vi "NI Analog.vi"(8 "error in (no error)":errorcluster, 11 "Message Queues":T1) -> (0 "error out":errorcluster, 3 "Message Queue out":refnum<queue>)   [LabVIEW 2014]
uses:
  support/Message Queue/All Message Queues.ctl
  support/Message Queue/Message Cluster.ctl
  Analog data.ctl
  Analog Input Cluster.ctl
  Analog Result Cluster.ctl
  <vilib>/DAQmx/write.llb/DAQmx Write (Analog DBL 1Chan 1Samp).vi
  <vilib>/DAQmx/read.llb/DAQmx Read (Analog 1D DBL 1Chan NSamp).vi
  <vilib>/DAQmx/read.llb/DAQmx Read (Analog 2D DBL NChan NSamp).vi
  support/Message Queue/Enqueue Message (Single).vi
  <vilib>/DAQmx/miscellaneous.llb/DAQmx Fill In Error Info.vi
  support/Message Queue/Lossy Enqueue Message (Single).vi
  <vilib>/Utility/error.llb/Error Cluster From Error Code.vi
  <vilib>/ErrorRing/Error Ring.xnode
  support/Message Queue/Message Queue.lvlib
panel:
  out "Port Write Time [ms] 2":u32
  out "Port Write Time [ms]":u32
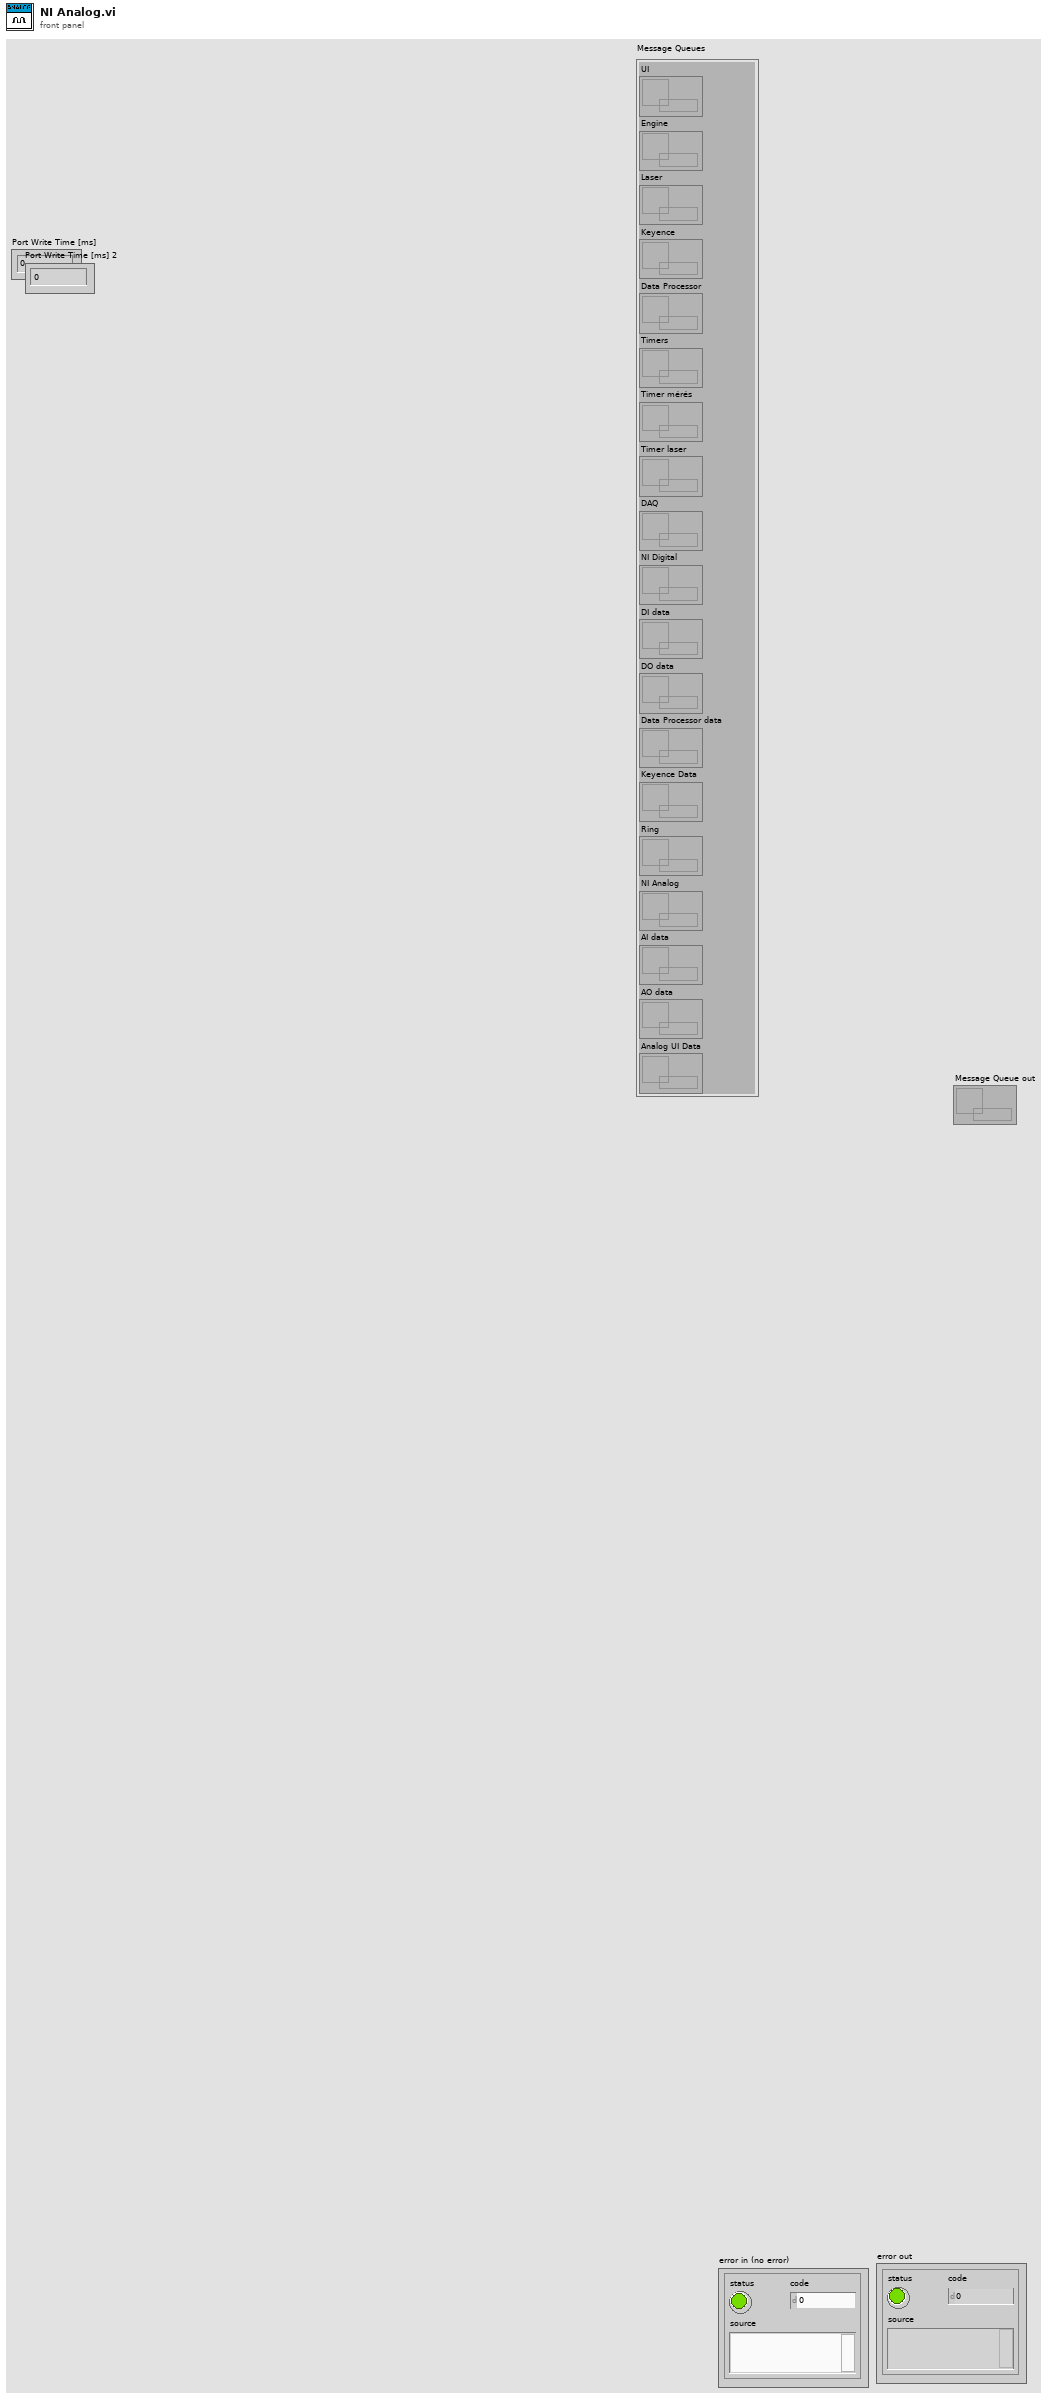
[diagram p1: front panel]
types:
  T1 = typedef "Message Queue.lvlib/All Message Queues.ctl" = cluster{"UI":refnum<queue>, "Engine":refnum<queue>, "Laser":refnum<queue>, "Keyence":refnum<queue>, "Data Processor":refnum<queue>, "Timers":refnum<queue>, "Timer mérés":refnum<queue>, "Timer laser":refnum<queue>, "DAQ":refnum<queue>, "NI Digital":refnum<queue>, "DI data":refnum<queue>, "DO data":refnum<queue>, "Data Processor data":refnum<queue>, "Keyence Data":refnum<queue>, "Ring":refnum<queue>, "NI Analog":refnum<queue>, "AI data":refnum<queue>, "AO data":refnum<queue>, "Analog UI Data":refnum<queue>}
  T2 = typedef "Analog data.ctl" = cluster{"URref":refnum<k21>, "UR":refnum<k21>, "UNTC":refnum<k21>, "UISOL":refnum<k21>, "TEMP":refnum<k21>, "dUref":refnum<k21>, "dU_":refnum<k21>, "UCTRL":refnum<k21>, "U48":refnum<k21>, "NI analog":refnum<k21>}
  T3 = typedef "Analog Input Cluster.ctl" = cluster{"NI-6221":cluster{"Sensor":dbl, "Uref":dbl, "Temperature":dbl, "Uisol":dbl, "NTC":dbl, "U48":dbl, "U15":dbl}, "Analog Result":T4, "AI engedélyezés":bool, "dU":dbl[]}
  T4 = typedef "Analog Result Cluster.ctl" = cluster{"Szenzor ellenállás":dbl, "NTC ellenállás":dbl, "Szigetelési ellenállás":dbl, "Hõmérséklet":dbl, "48V":dbl, "15V":dbl, "Elvárt NTC ellenállás":dbl, "Számolt NTC hõmérséklet":dbl}
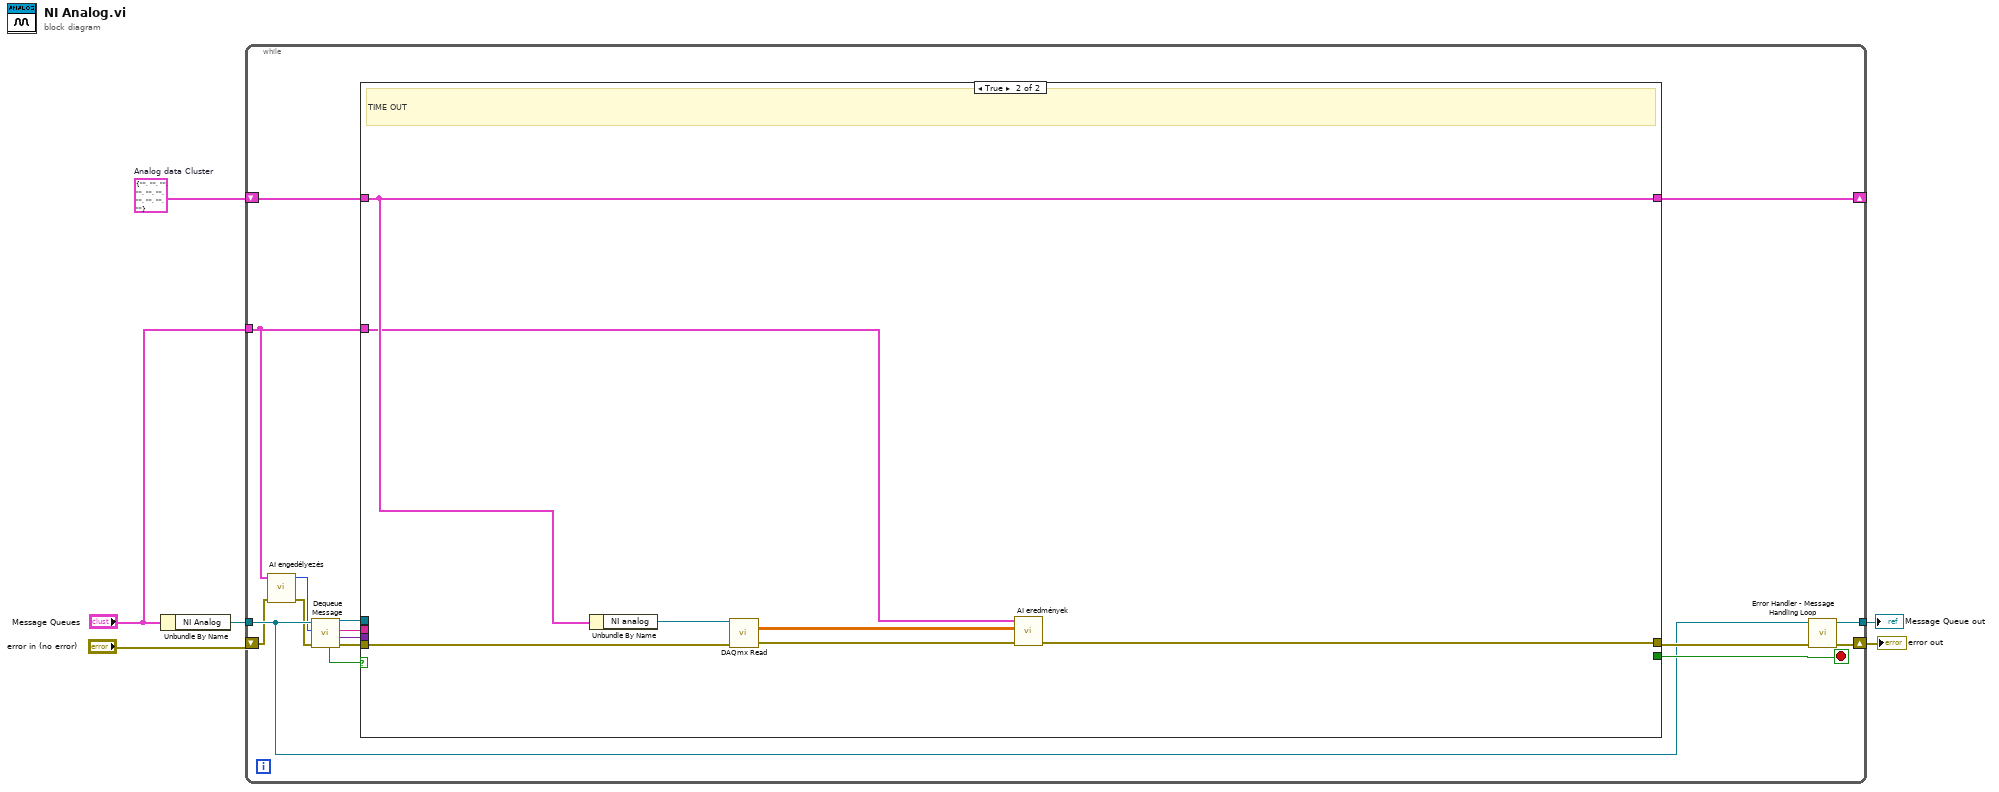
[diagram p0: block diagram]
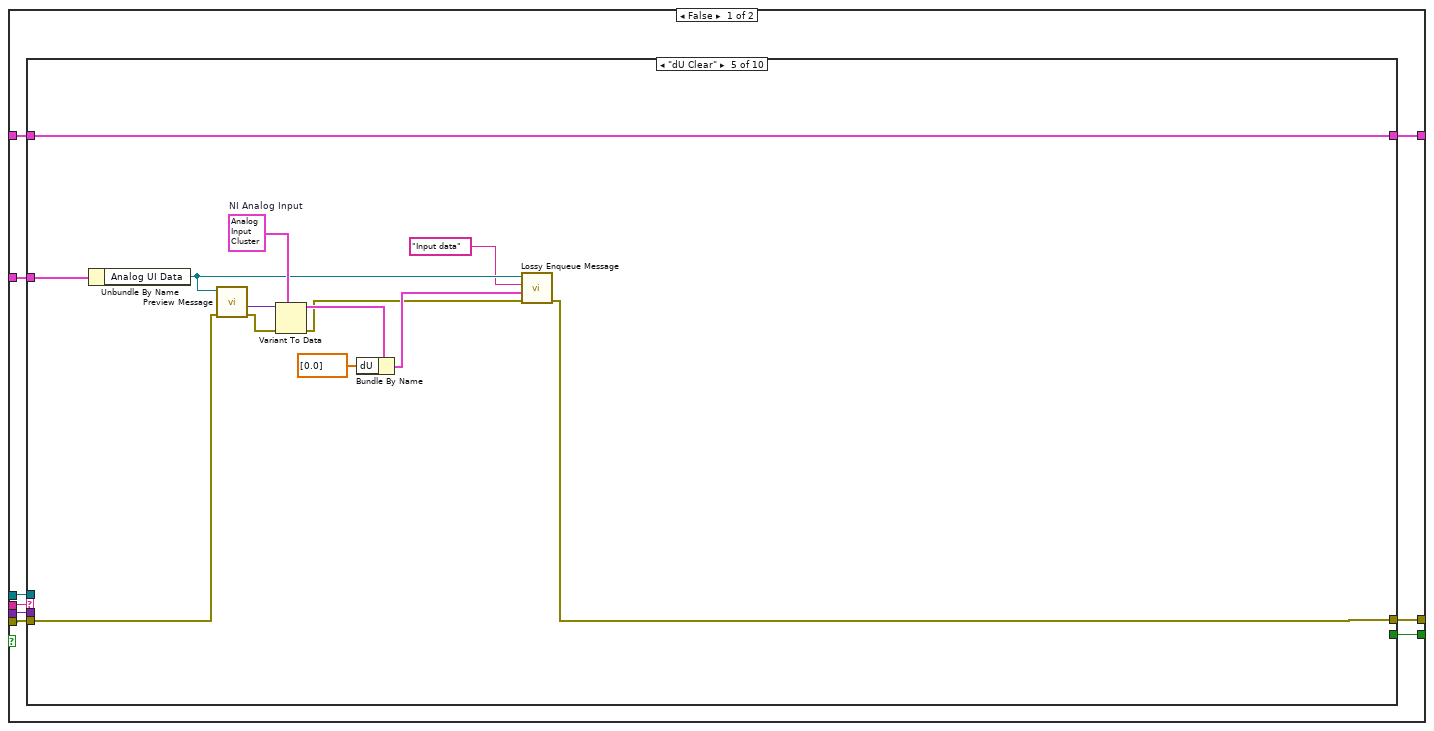
[diagram p2: hidden frame]
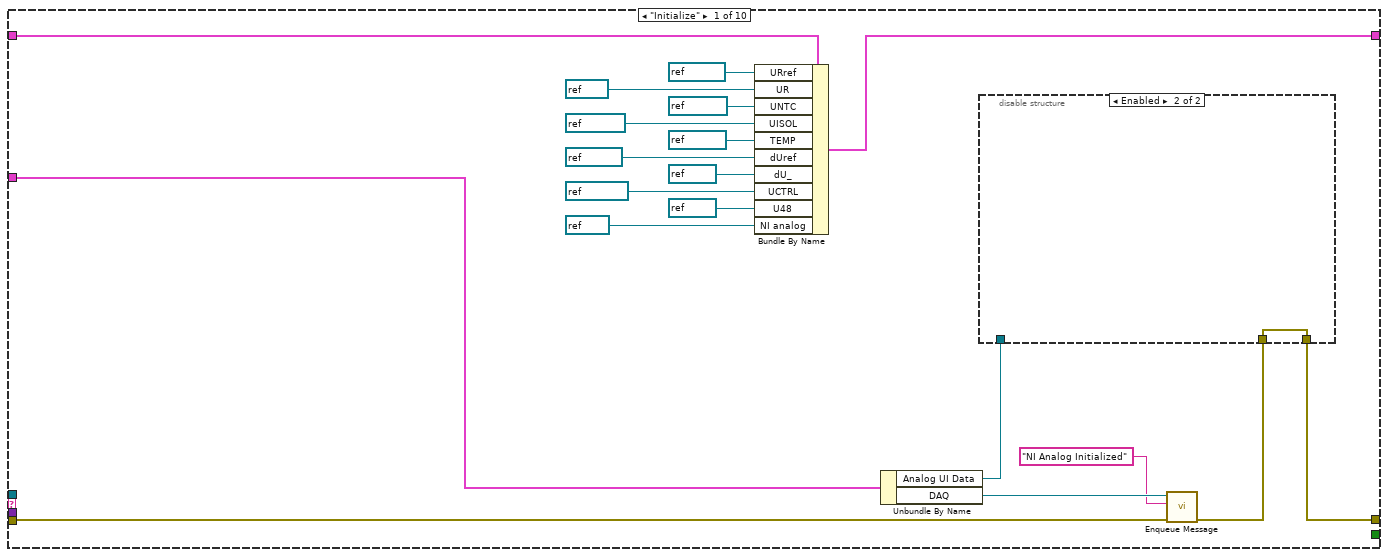
[diagram p3: hidden frame]
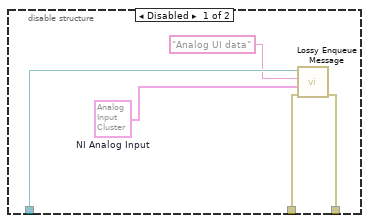
[diagram p4: hidden frame]
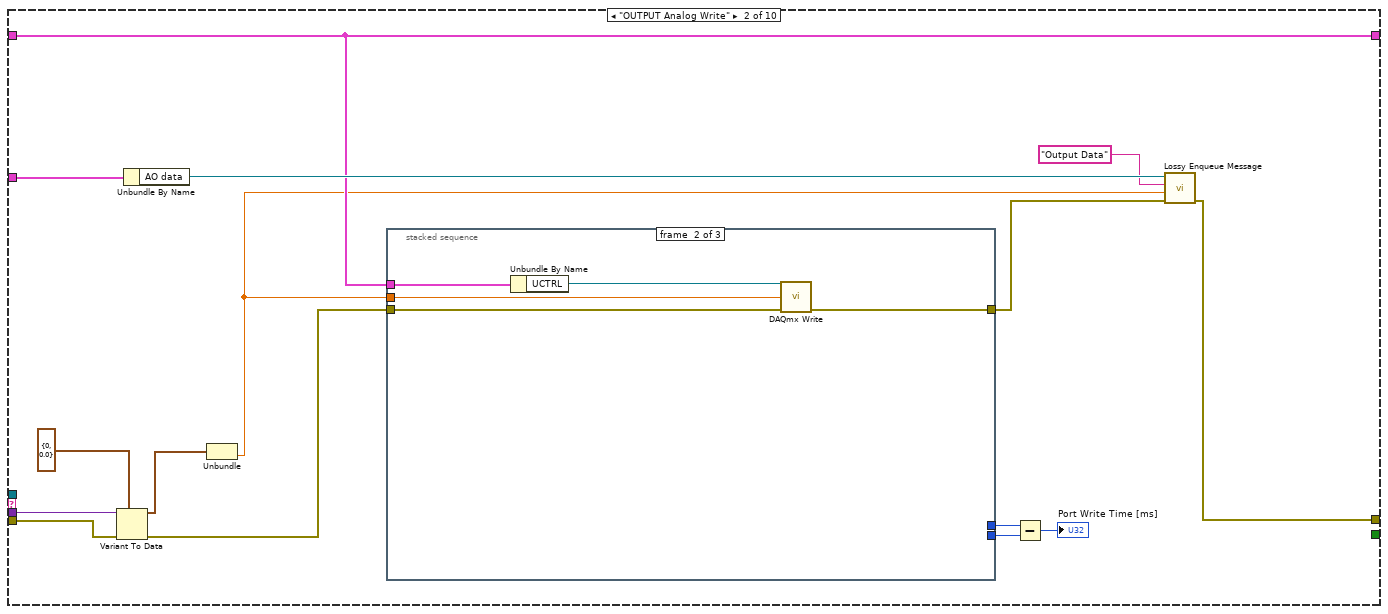
[diagram p5: hidden frame]
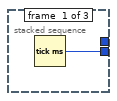
[diagram p6: hidden frame]
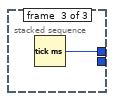
[diagram p7: hidden frame]
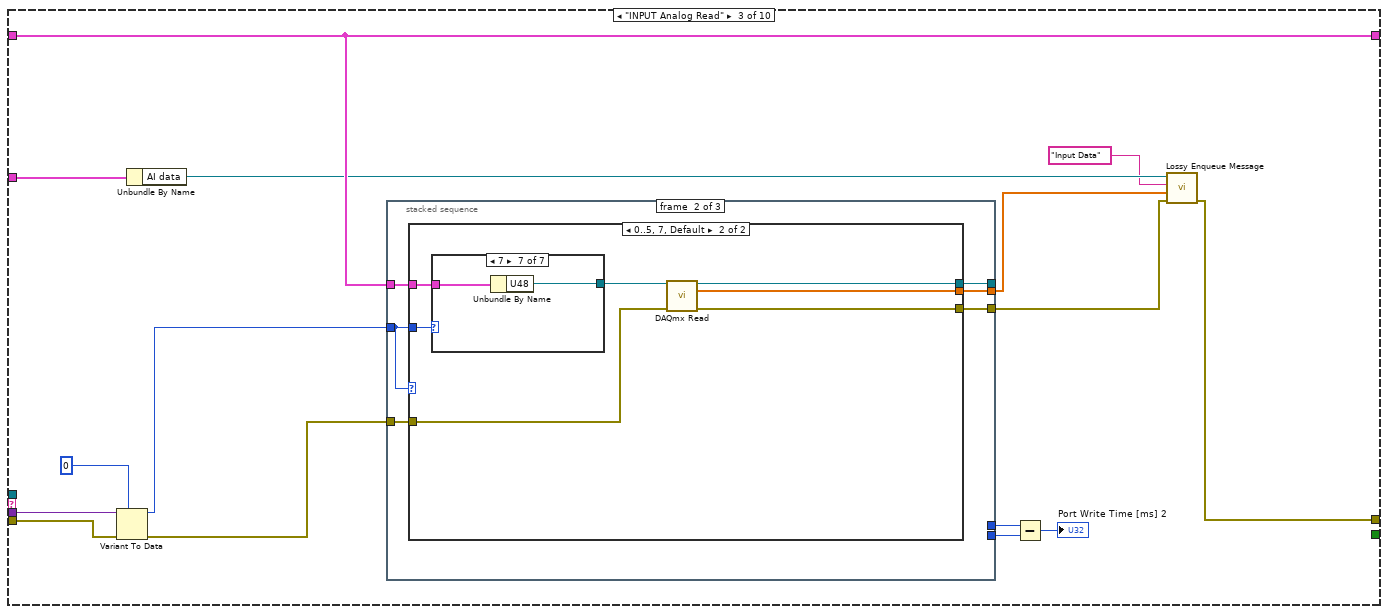
[diagram p8: hidden frame]
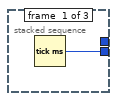
[diagram p9: hidden frame]
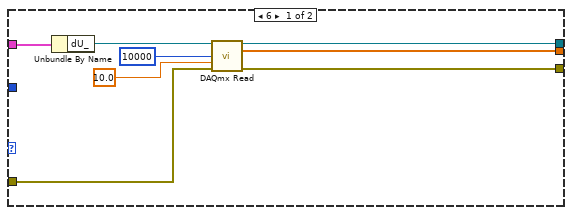
[diagram p10: hidden frame]
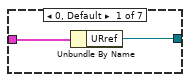
[diagram p11: hidden frame]
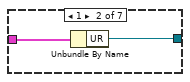
[diagram p12: hidden frame]
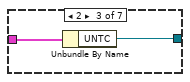
[diagram p13: hidden frame]
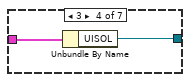
[diagram p14: hidden frame]
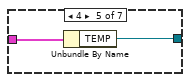
[diagram p15: hidden frame]
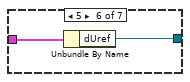
[diagram p16: hidden frame]
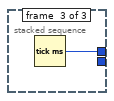
[diagram p17: hidden frame]
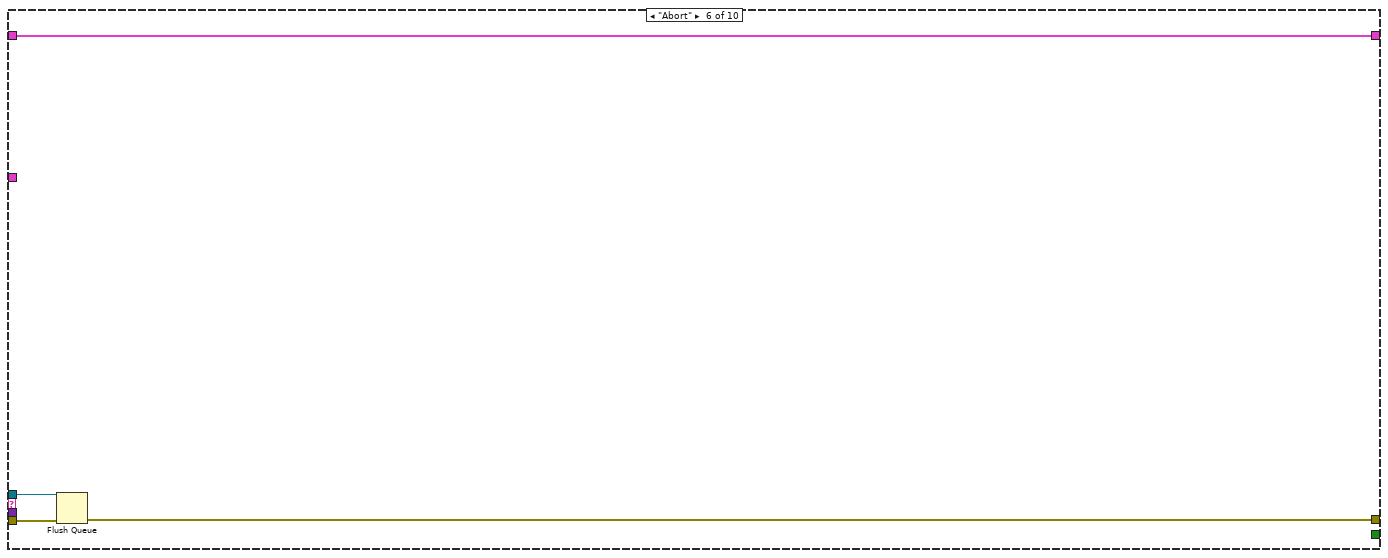
[diagram p19: hidden frame]
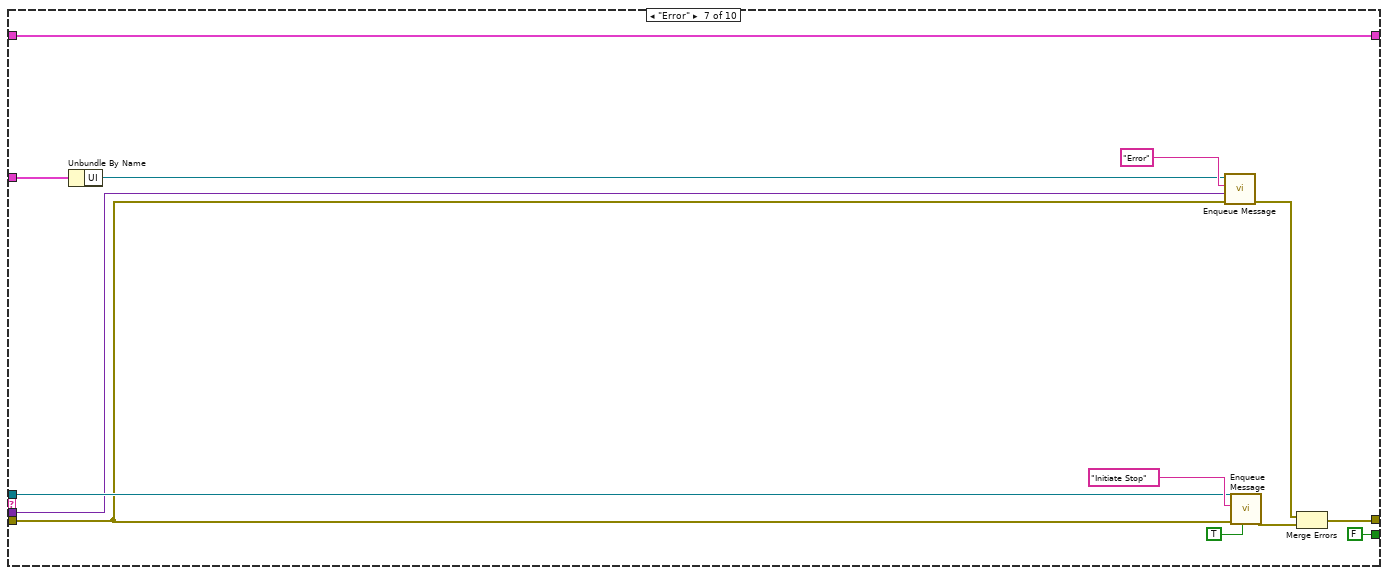
[diagram p20: hidden frame]
diagram:
  w1 = T2 {"URref"="", "UR"="", "UNTC"="", "UISOL"="", "TEMP"="", "dUref"="", "dU_"="", "UCTRL"="", "U48"="", "NI analog"=""}  # Analog data Cluster
  n1 = Unbundle By Name("Message Queues") -> ("NI Analog"=w3:refnum<queue>)
  n2 = while {
    tunnel: w3 -> [w14]
    shift-right: [w12] -> _
    shift-left: w1 -> [w18]
    shift-right: [w16] -> w6
    shift-left: "error in (no error)" -> [w9]
    tunnel: "Message Queues" -> [w10]
    tunnel: [w13] -> w2
    stop <- w20 stop-if-true
    n3 = call "AI engedélyezés.vi"("error in (no error)"=w9, "Message Queues"=w10) -> ("error out"=w8:errorcluster, "timeout in ms (-1)"=w7:i32)  [unwired: 8 in]
    n4 = call "Dequeue Message.vi"("error in (no error)"=w8, "timeout in ms (-1)"=w7, "Message Queue"=w14) -> ("error out"=w22:errorcluster, "Message Data"=w17:variant, "Message"=w11:string, "dup Message Queue"=w21:refnum<queue>, "timed out?"=w19:bool)  [unwired: 4 in]
    n5 = case shown="True" w19 {
      tunnel: w11 -> [w31 _]
      tunnel: w22 -> [w30 w198]
      tunnel: w21 -> [w29 _]
      tunnel: [w28 _] -> w20
      tunnel: [w27 w197] -> w15
      tunnel: w18 -> [w25 w200]
      tunnel: [w26 w200] -> w12
      tunnel: w17 -> [w24 _]
      tunnel: w10 -> [w23 w195]
      frame False {
        n6 = case shown="\"dU Clear\"" w31 {
          selector: w31 -> [_ _ _ _ _ _ _ _ _ w184]
          tunnel: w30 -> [w32 w64 w90 w131 w134 w147 w152 w164 w177 _]
          tunnel: w29 -> [_ _ _ _ _ w149 w159 w166 w183 _]
          tunnel: [w34 w58 w82 w131 w133 w146 w153 w167 w175 w185] -> w27
          tunnel: [_ _ _ _ _ _ FALSE _ TRUE _] -> w28
          tunnel: [w36 w61 w87 w132 w145 w148 w161 w163 w181 w186] -> w26
          tunnel: w25 -> [w33 w61 w87 w132 w145 w148 w161 w163 w181 w186]
          tunnel: w24 -> [_ w63 w89 _ _ _ w151 _ _ _]
          tunnel: w23 -> [w50 w62 w88 _ w144 _ w158 _ w176 _]
          frame "Initialize" {
            n7 = Bundle By Name(cluster=w33, "URref"=refnum<k21> "URref" ("UR"), "UR"=refnum<k21> "UR", "UNTC"=refnum<k21> "UNTC" ("UR"), "UISOL"=refnum<k21> "UISOL" ("UR"), "TEMP"=refnum<k21> "TEMP" ("UR"), "dUref"=refnum<k21> "dUref" ("UR"), "dU_"=refnum<k21> "dU_" ("UR"), "UCTRL"=refnum<k21> "UCTRL" ("task/channels in"), "U48"=refnum<k21> "U48" ("UR"), "NI analog"=refnum<k21> "AI_" ("UR")) -> (w36:T2)
            n8 = Unbundle By Name(w50) -> ("Analog UI Data"=w37:refnum<queue>, "DAQ"=w49:refnum<queue>)
            n9 = call-poly "Enqueue Message.vi"("error in (no error)"=w32, "Message"="NI Analog Initialized", "Message Queue"=w49) -> ("error out"=w35:errorcluster)  [unwired: 7 in, 1 out]
            n10 = disable-structure shown="Enabled" {
              disable-tunnel: w37 -> [w55 _]
              disable-tunnel: w35 -> [w54 w56]
              disable-tunnel: [w53 w56] -> w34
              frame Disabled {
                w51 = T3 {"NI-6221"={"Sensor"=0.0, "Uref"=0.0, "Temperature"=0.0, "Uisol"=0.0, "NTC"=0.0, "U48"=0.0, "U15"=0.0}, "Analog Result"={"Szenzor ellenállás"=0.0, "NTC ellenállás"=0.0, "Szigetelési ellenállás"=0.0, "Hõmérséklet"=0.0, "48V"=0.0, "15V"=0.0, "Elvárt NTC ellenállás"=0.0, "Számolt NTC hõmérséklet"=0.0}, "AI engedélyezés"=FALSE, "dU"=[]}  # NI Analog Input
                n11 = call-poly "Lossy Enqueue Message.vi"("error in (no error)"=w54, "Message Data"=w51, "Message"="Analog UI data", "Message Queue"=w55) -> ("error out"=w53:errorcluster)  [unwired: 6 in, 1 out]
              }
              frame Enabled {
              }
            }
          }
          frame "OUTPUT Analog Write" {
            n12 = Variant To Data(error in=w64, type=cluster{i32, "UCtrl":dbl} {0, "UCtrl"=0.0} ("cluster"), Variant=w63) -> (data=w59:cluster{i32, "UCtrl":dbl}, error out=w66:errorcluster)
            n13 = Unbundle By Name(w62) -> ("AO data"=w71:refnum<queue>)
            n14 = Unbundle(w59) -> ("UCtrl"=w57:dbl)  [unwired: 1 out]
            n15 = stacked-sequence {
              tunnel: w66 -> [_ w74 _]
              tunnel: [w72 _ _] -> w68
              tunnel: [_ _ w78] -> w67
              tunnel: w61 -> [_ w77 _]
              tunnel: [_ w75 _] -> w65
              tunnel: w57 -> [_ w73 _]
              frame #0 {
                n16 = Tick Count (ms)() -> (millisecond timer value=w72:u32)
              }
              frame #1 {
                n17 = Unbundle By Name(w77) -> ("UCTRL"=w76:refnum<k21>)
                n18 = call-poly <vilib>:"DAQmx Write.vi"("task/channels in"=w76, "data"=w73, "error in"=w74) -> ("error out"=w75:errorcluster)  [unwired: 10 in, 2 out]
              }
              frame #2 {
                n19 = Tick Count (ms)() -> (millisecond timer value=w78:u32)
              }
            }
            n20 = Subtract(x=w67, y=w68) -> (x-y=→"Port Write Time [ms]":u32)
            n21 = call-poly "Lossy Enqueue Message.vi"("error in (no error)"=w65, "Message Data"=w57, "Message"="Output Data", "Message Queue"=w71) -> ("error out"=w58:errorcluster)  [unwired: 6 in, 1 out]
          }
          frame "INPUT Analog Read" {
            n22 = Variant To Data(error in=w90, type=u32 0, Variant=w89) -> (data=w80:u32, error out=w79:errorcluster)
            n23 = Unbundle By Name(w88) -> ("AI data"=w86:refnum<queue>)
            n24 = stacked-sequence {
              tunnel: w79 -> [_ w99 _]
              tunnel: [w94 _ _] -> w92
              tunnel: [_ _ w130] -> w91
              tunnel: w87 -> [_ w100 _]
              tunnel: w80 -> [_ w97 _]
              tunnel: [_ w98 _] -> w83
              tunnel: [_ w96 _] -> w84
              tunnel: [_ w95 _] -> _
              frame #0 {
                n25 = Tick Count (ms)() -> (millisecond timer value=w94:u32)
              }
              frame #1 {
                n26 = case shown="0..5, 7, Default" w97 {
                  tunnel: w100 -> [w108 w115]
                  tunnel: w97 -> [_ w114]
                  tunnel: w99 -> [w106 w112]
                  tunnel: [w102 w111] -> w96
                  tunnel: [w105 w110] -> w98
                  tunnel: [w101 w109] -> w95
                  frame 6 {
                    n27 = Unbundle By Name(w108) -> ("dU_"=w107:refnum<k21>)
                    n28 = call-poly <vilib>:"DAQmx Read.vi"("task/channels in"=w107, "number of samples per channel"=10000, "timeout"=10.0, "error in"=w106) -> ("task out"=w101:refnum<k21>, "data"=w102:dbl[], "error out"=w105:errorcluster)  [unwired: 9 in]
                  }
                  frame 0..5, 7, Default {
                    n29 = case shown="7" w114 {
                      tunnel: w115 -> [w117 w119 w121 w123 w125 w127 w129]
                      tunnel: [w116 w118 w120 w122 w124 w126 w128] -> w113
                      frame 0, Default {
                        n30 = Unbundle By Name(w117) -> ("URref"=w116:refnum<k21>)
                      }
                      frame 1 {
                        n31 = Unbundle By Name(w119) -> ("UR"=w118:refnum<k21>)
                      }
                      frame 2 {
                        n32 = Unbundle By Name(w121) -> ("UNTC"=w120:refnum<k21>)
                      }
                      frame 3 {
                        n33 = Unbundle By Name(w123) -> ("UISOL"=w122:refnum<k21>)
                      }
                      frame 4 {
                        n34 = Unbundle By Name(w125) -> ("TEMP"=w124:refnum<k21>)
                      }
                      frame 5 {
                        n35 = Unbundle By Name(w127) -> ("dUref"=w126:refnum<k21>)
                      }
                      frame 7 {
                        n36 = Unbundle By Name(w129) -> ("U48"=w128:refnum<k21>)
                      }
                    }
                    n37 = call-poly <vilib>:"DAQmx Read.vi"("task/channels in"=w113, "error in"=w112) -> ("task out"=w109:refnum<k21>, "data"=w111:dbl[], "error out"=w110:errorcluster)  [unwired: 11 in]
                  }
                }
              }
              frame #2 {
                n38 = Tick Count (ms)() -> (millisecond timer value=w130:u32)
              }
            }
            n39 = Subtract(x=w91, y=w92) -> (x-y=→"Port Write Time [ms] 2":u32)
            n40 = call-poly "Lossy Enqueue Message.vi"("error in (no error)"=w83, "Message Data"=w84, "Message"="Input Data", "Message Queue"=w86) -> ("error out"=w82:errorcluster)  [unwired: 6 in, 1 out]
          }
          frame "Refresh" {
            # "A Time Out érték változtatása miatt egyszer frissíteni kell a Queue-t, hogy érvényre jusson a változtatás."
          }
          frame "dU Clear" {
            w142 = T3 {"NI-6221"={"Sensor"=0.0, "Uref"=0.0, "Temperature"=0.0, "Uisol"=0.0, "NTC"=0.0, "U48"=0.0, "U15"=0.0}, "Analog Result"={"Szenzor ellenállás"=0.0, "NTC ellenállás"=0.0, "Szigetelési ellenállás"=0.0, "Hõmérséklet"=0.0, "48V"=0.0, "15V"=0.0, "Elvárt NTC ellenállás"=0.0, "Számolt NTC hõmérséklet"=0.0}, "AI engedélyezés"=FALSE, "dU"=[]}  # NI Analog Input
            n41 = Unbundle By Name(w144) -> ("Analog UI Data"=w139:refnum<queue>)
            n42 = call "Preview Message.vi"("error in (no error)"=w134, "Message Queue"=w139) -> ("error out"=w136:errorcluster, "Message Data"=w143:variant)  [unwired: 5 in, 3 out]
            n43 = Variant To Data(error in=w136, type=w142, Variant=w143) -> (data=w141:T3, error out=w135:errorcluster)
            n44 = Bundle By Name(cluster=w141, "dU"=dbl[] [0.0]) -> (w138:T3)
            n45 = call-poly "Lossy Enqueue Message.vi"("error in (no error)"=w135, "Message Data"=w138, "Message"="Input data", "Message Queue"=w139) -> ("error out"=w133:errorcluster)  [unwired: 6 in, 1 out]
          }
          frame "Abort" {
            n46 = Flush Queue(queue=w149, error in (no error)=w147) -> (error out=w146:errorcluster)  [unwired: 2 out]
          }
          frame "Error" {
            n47 = Unbundle By Name(w158) -> ("UI"=w156:refnum<queue>)
            n48 = call-poly "Enqueue Message.vi"("error in (no error)"=w152, "Message Data"=w151, "Message"="Error", "Message Queue"=w156) -> ("error out"=w154:errorcluster)  [unwired: 6 in, 1 out]
            n49 = call-poly "Enqueue Message.vi"("Priority Message? (F)"=TRUE, "error in (no error)"=w152, "Message"="Initiate Stop", "Message Queue"=w159) -> ("error out"=w155:errorcluster)  [unwired: 6 in, 1 out]
            n50 = Merge Errors(w154, w155) -> (w153:errorcluster)
          }
          frame "Initiate Stop" {
            n51 = call-poly "Enqueue Message.vi"("Priority Message? (F)"=TRUE, "error in (no error)"=w164, "Message"="Program Stop", "Message Queue"=w166) -> ("error out"=w167:errorcluster)  [unwired: 6 in, 1 out]
          }
          frame "Program Stop" {
            n52 = Flush Queue(queue=w183, error in (no error)=w177) -> (error out=w174:errorcluster)  [unwired: 2 out]
            n53 = Unbundle By Name(w176) -> ("AI data"=w171:refnum<queue>, "AO data"=w178:refnum<queue>)
            n54 = Flush Queue(queue=w178, error in (no error)=w177) -> (queue out=w179:refnum<queue>, error out=w180:errorcluster)  [unwired: 1 out]
            n55 = Release Queue(queue=w179, error in (no error)=w180) -> (error out=w170:errorcluster)  [unwired: 1 in, 2 out]
            n56 = Flush Queue(queue=w171, error in (no error)=w170) -> (queue out=w173:refnum<queue>, error out=w172:errorcluster)  [unwired: 1 out]
            n57 = Release Queue(queue=w173, error in (no error)=w172) -> (error out=w169:errorcluster)  [unwired: 1 in, 2 out]
            n58 = Merge Errors(w169, w174) -> (w175:errorcluster)
          }
          frame Default {
            n59 = xnode "Error Ring"("parameter 0"=w184) -> ("error out"=w185:errorcluster)
          }
        }
      }
      frame True {
        # "TIME OUT"
        n60 = Unbundle By Name(w200) -> ("NI analog"=w199:refnum<k21>)
        n61 = call-poly <vilib>:"DAQmx Read.vi"("task/channels in"=w199, "error in"=w198) -> ("data"=w194:dbl[][], "error out"=w196:errorcluster)  [unwired: 11 in, 1 out]
        n62 = call "AI eredmények.vi"("error in (no error)"=w196, "data"=w194, "Message Queues"=w195) -> ("error out"=w197:errorcluster)  [unwired: 8 in]
      }
    }
    n63 = call "Error Handler - Message Handling Loop.vi"("error in (no error)"=w15, "Message Queue"=w14) -> ("dup error in"=w16:errorcluster, "dup Message Queue"=w13:refnum<queue>)  [unwired: 8 in]
  }
  "error out" <- w6
  "Message Queue out" <- w2
